vi "Offset timestamps in file.vi"() -> ()   [LabVIEW 2017]
uses:
  <vilib>/Utility/file.llb/Write To Spreadsheet File (I64).vi
panel:
  out "all rows":i64[][](array[numeric])
  in  "Offset":i64
  in  "Function":T1(ring)
  out "Rel. time":i64[](array[numeric])
  in  "Cam video timestamp file":path=path "C:/Users/All Other Users/Desktop/theo_videos/150610_15_33_59/150610_15_33_59 VidRec/10-06-2015 15_45_07-EyeCam-relative times.txt"
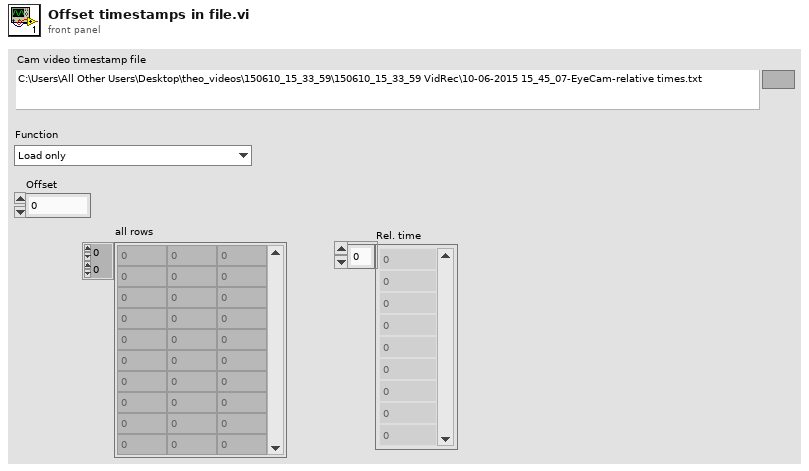
[diagram p1: front panel]
types:
  T1 = enum16{"Load only", "Load and offset only", "Load, offset and save back to the file"}
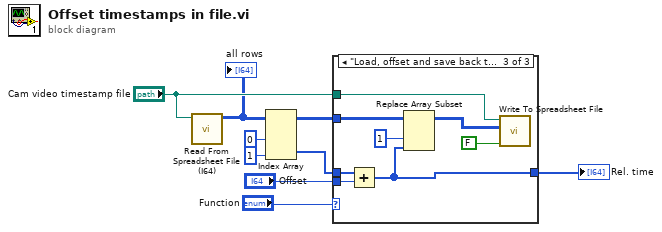
[diagram p0: block diagram]
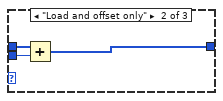
[diagram p3: hidden frame]
diagram:
  n1 = call <vilib>:"Read From Spreadsheet File (I64).vi"("file path (dialog if empty)"="Cam video timestamp file") -> ("all rows"=w1:i64[][])  [unwired: 6 in, 4 out]
  "all rows" <- w1
  n2 = Index Array(array=w1, index (col) #1=0 ("disabled index (col)"), index (col) #2=1 ("index (row)")) -> (element #2=w6:i64[])  [unwired: 2 in, 1 out]
  n3 = case shown="\"Load, offset and save back to the file\"" "Function" {
    tunnel: w6 -> [w9 w12 w20]
    tunnel: "Offset" -> [_ w11 w19]
    tunnel: [w9 w10 w15] -> w3
    tunnel: "Cam video timestamp file" -> [_ _ w18]
    tunnel: w1 -> [_ _ w17]
    frame "Load only", Default {
    }
    frame "Load and offset only" {
      n4 = Add(x=w12, y=w11) -> (x+y=w10:i64[])
    }
    frame "Load, offset and save back to the file" {
      n5 = Add(x=w20, y=w19) -> (x+y=w15:i64[])
      n6 = Replace Array Subset(array=w17, new element=w15, index (col)=1 ("disabled index (col)")) -> (w13:i64[][])  [unwired: 1 in]
      n7 = call-poly <vilib>:"Write To Spreadsheet File.vi"("append to file? (new file:F)"=FALSE, "2D data"=w13, "file path (dialog if empty)"=w18) -> ()  [unwired: 5 in, 1 out]
    }
  }
  "Rel. time" <- w3
